vi "fgt create simulated instr.vi"(6 "version":u16 caption="version (default)", 8 "error in (no error)":errorcluster, 9 "config":i32[](array[numeric]), 10 "SN":u16, 11 "Type":T1) -> (0 "error out":errorcluster)   [LabVIEW 2016, in "fgt_SDK.lvlib"]
doc: "Creates a simulated Fluigent instrument, which can be detected and initialized like a real one, for the purposes of testing and demonstrations.\nThe version input can usually be left disconnected to use the default firmware version for the specified instrument type.\nSee the user manual for help on how to construct the config array to specify the instrument's configuration."
uses:
  fgt_SDK.lvlib
  TypeDefs/fgt_INSTRUMENT_TYPE.ctl
  dlls/fgt_SDK_32.dll
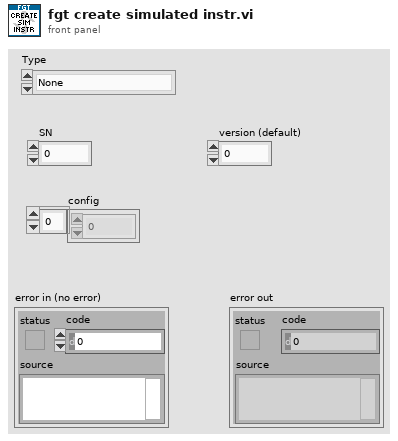
[diagram p1: front panel]
types:
  T1 = typedef "fgt_SDK.lvlib/fgt_INSTRUMENT_TYPE.ctl" = enum32{"None", "MFCS", "MFCS_EZ", "FRP", "LineUP", "IPS"}
  T2 = typedef "fgt_SDK.lvlib/fgt_STATUS_INFO.ctl" = cluster{"InstrType":T1, "instrSN":u16, "errorCode":u8, "infoCode":u8, "detail":string}
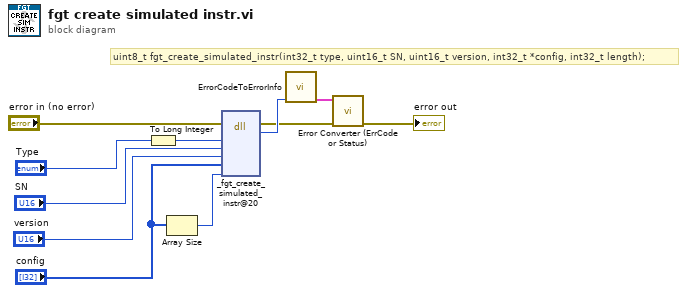
[diagram p0: block diagram]
diagram:
  # "uint8_t fgt_create_simulated_instr(int32_t type, uint16_t SN, uint16_t version, int32_t *config, int32_t length);"
  n1 = To Long Integer(number="Type") -> (32bit integer=w6:i32)
  n2 = Array Size(array="config") -> (size(s)=w3:i32)
  n3 = dll-call lib="C:/projects/SDK/fgt-sdk-labview/dlls/fgt_SDK_*.*" fn="_fgt_create_simulated_instr@20"(error in="error in (no error)", "type"=w6, "SN"="SN", "version"="version", "config"="config", "length"=w3) -> (error out=w8:errorcluster, "return type"=w9:u8)  [unwired: 7 in, 1 out]
  n4 = call "ErrorCodeToErrorInfo.vi"("return type"=w9) -> ("StatusInfo"=w10:T2)  [unwired: 10 in]
  n5 = call "Error Converter (ErrCode or Status).vi"("error in (no error)"=w8, "StatusInfo"=w10) -> ("error out"=→"error out":errorcluster)  [unwired: 9 in]
